vi "Save_incrementally_171213.vi"(0 "Temporary file output path":path, 1 "Play / Pause":bool, 2 "Sensor read input":sgl[][](array[numeric]), 5 "Loop iteration":i32, 7 "Loop speed in ms":u16, 9 "Save every N seconds":u32=15, 11 "error in (no error)":errorcluster) -> (4 "Eff. save interval":sgl, 15 "error out":errorcluster)   [LabVIEW 2016]
uses:
  <vilib>/Utility/file.llb/Write Delimited Spreadsheet (DBL).vi
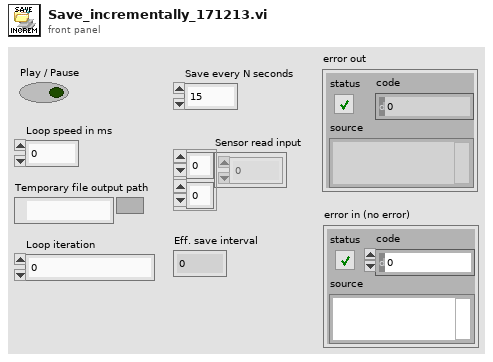
[diagram p1: front panel]
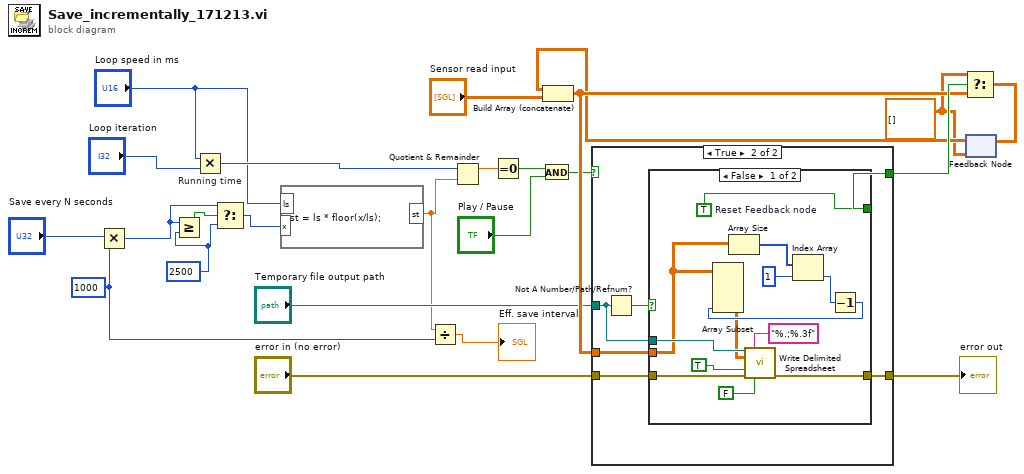
[diagram p0: block diagram]
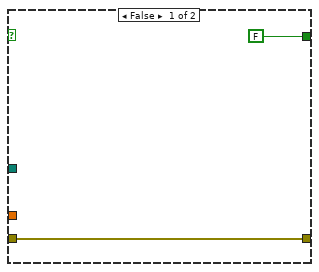
[diagram p2: hidden frame]
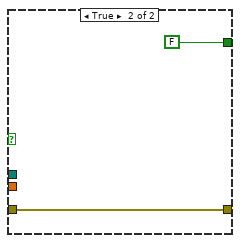
[diagram p3: hidden frame]
diagram:
  w1 = u32 1000 ("y")
  w8 = 2500
  w12 = sgl[][] []
  n1 = Multiply(x="Save every N seconds", y=w1) -> (x*y=w4:u32)
  n2 = Greater Or Equal?(x=w4, y=w8) -> (x >= y?=w9:bool)
  n3 = Multiply "Running time"(x="Loop speed in ms", y="Loop iteration") -> (x*y=w16:i32)
  n4 = Select(t=w4, s=w9, f=w8) -> (s? t:f=w6:u32)
  n5 = formula code="st = ls * floor(x/ls);"("ls"="Loop speed in ms", "x"=w6) -> ("st"=w3:dbl)
  n6 = Divide(x=w3, y=w1) -> (x/y=→"Eff. save interval":dbl)
  n7 = Quotient & Remainder(x=w16, y=w3) -> (x-y*floor(x/y)=w14:dbl)  [unwired: 1 out]
  n8 = Equal To 0?(x=w14) -> (x = 0?=w15:bool)
  n9 = And(x=w15, y="Play / Pause") -> (x .and. y?=w20:bool)
  n10 = feedback #1(w12) -> (w21:sgl[][])
  n11 = Build Array (concatenate)(w21, "Sensor read input") -> (w22:sgl[][])
  n12 = case shown="True" w20 {
    tunnel: "Temporary file output path" -> [_ w31]
    tunnel: w22 -> [_ w30]
    tunnel: [FALSE w29] -> w24
    tunnel: "error in (no error)" -> [w25 w28]
    tunnel: [w25 w27] -> w10
    frame False {
    }
    frame True {
      n13 = Not A Number/Path/Refnum?(number/path/refnum=w31) -> (NaN/Path/Refnum?=w32:bool)
      n14 = case shown="False" w32 {
        tunnel: w31 -> [w45 _]
        tunnel: w30 -> [w37 _]
        tunnel: [w42 FALSE] -> w29
        tunnel: w28 -> [w41 w46]
        tunnel: [w40 w46] -> w27
        frame False {
          w42 = TRUE  # Reset Feedback node
          n15 = Array Size(array=w37) -> (size(s)=w39:i32[])
          n16 = Index Array(array=w39, index=1) -> (element=w36:i32)
          n17 = Decrement(x=w36) -> (x-1=w35:i32)
          n18 = Array Subset(array=w37, length (col)=w35) -> (w34:sgl[][])  [unwired: 3 in]
          n19 = call-poly <vilib>:"Write Delimited Spreadsheet.vi"("file path (dialog if empty)"=w45, "format (%.3f)"="%.;%.3f", "2D data"=w34, "append to file? (new file:F)"=TRUE, "error in (no error)"=w41, "transpose? (no:F)"=FALSE) -> ("error out"=w40:errorcluster)  [unwired: 8 in, 1 out]
        }
        frame True {
        }
      }
    }
  }
  "error out" <- w10
  n20 = Select(t=w12, s=w24, f=w22) -> (s? t:f=w23:sgl[][])
  n21 = feedback-in #1(w23) -> ()
